vi "Test-wheel-Params.vi"() -> ()   [LabVIEW 2019]
uses:
  ShootDualTalonSRX/Dist_Type.ctl
  ShootDualTalonSRX/Time_Units_Control.ctl
  ShootDualTalonSRX/ShootDualTalonSRX_Motor_Pair.lvlib
panel:
  out "Ft/Sec":dbl
  out "Feet":dbl
  out "Counts/.1Sec":dbl format="%.7f"
  out "Counts":dbl format="%.7f"
  in  "Feet/Sec":dbl
  in  "Feet":dbl
  out "Units":string
  in  "Time":T1
  in  "Enc Edges / Rev":dbl=1440.0 format="%.4f"
  in  "Wheel Radius In":dbl=3.0 format="%.4f"
  in  "Distance Type":T2
  out "VelUnits/Count in 0.1":dbl format="%.7f"
  out "Count/VelUnits In 0.1 SEC":dbl format="%.7f"
  out "Dist/Count":dbl format="%.7f"
  out "Count/Dist":dbl format="%.7f"
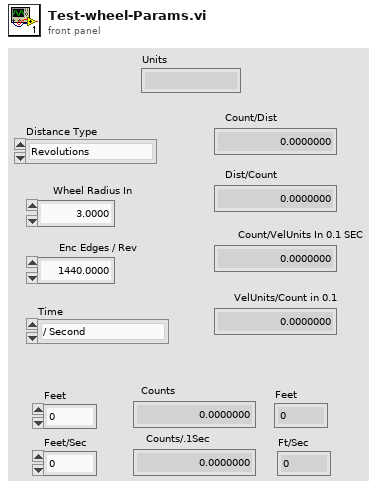
[diagram p1: front panel]
types:
  T1 = typedef "ShootDualTalonSRX_Motor_Pair.lvlib/Time_Units_Control.ctl" = enum16{"/ Second", "/ Minute"}
  T2 = typedef "ShootDualTalonSRX_Motor_Pair.lvlib/Dist_Type.ctl" = enum16{"Revolutions", "Feet"}
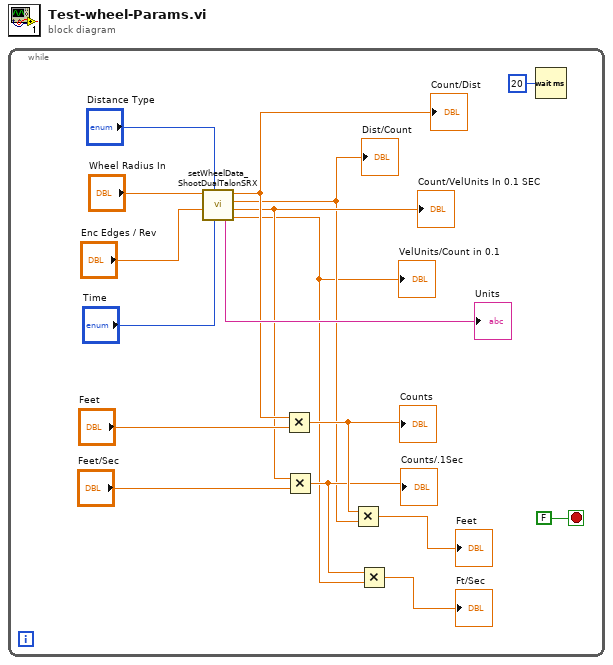
[diagram p0: block diagram]
diagram:
  n1 = while {
    stop <- FALSE stop-if-true
    n2 = call "setWheelData_ShootDualTalonSRX.vi"("Time"="Time", "Distance Type"="Distance Type", "Enc Edges / Rev"="Enc Edges / Rev", "Wheel Radius In"="Wheel Radius In") -> ("VelUnits/Count in 0.1"=w3:dbl, "Count/VelUnits In 0.1 SEC"=w7:dbl, "Dist/Count"=w4:dbl, "Count/Dist"=w8:dbl, "Units"=→"Units":string)  [unwired: 3 in]
    "Count/Dist" <- w8
    "Dist/Count" <- w4
    "Count/VelUnits In 0.1 SEC" <- w7
    "VelUnits/Count in 0.1" <- w3
    n3 = Multiply(x=w8, y="Feet") -> (x*y=w6:dbl)
    "Counts" <- w6
    n4 = Multiply(x=w7, y="Feet/Sec") -> (x*y=w5:dbl)
    "Counts/.1Sec" <- w5
    n5 = Multiply(x=w6, y=w4) -> (x*y=→"Feet":dbl)
    n6 = Multiply(x=w5, y=w3) -> (x*y=→"Ft/Sec":dbl)
    n7 = Wait (ms)(milliseconds to wait=u32 20) -> ()  [unwired: 1 out]
  }
